vi "Set FC1 ILC.vi"(10 "ilc":refnum<class "ILC.lvclass">, 11 "Model in":refnum<class "Model.lvclass">) -> (3 "Model out":refnum<class "Model.lvclass">)   [LabVIEW 2015, in "Model.lvclass"]
uses:
  Model.lvclass
  <userlib>/Common/ILC/ILC/ILC.lvclass
  Model.lvclass/Model.ctl
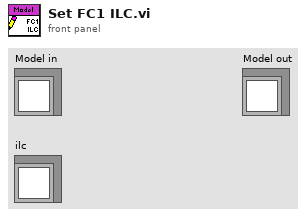
[diagram p1: front panel]
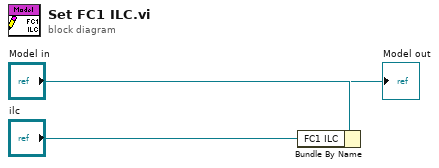
[diagram p0: block diagram]
diagram:
  n1 = Bundle By Name(cluster="Model in", "FC1 ILC"="ilc") -> (→"Model out":refnum<class "Model.lvclass">)
